vi "Archive Directory.vi"(8 "Error In":errorcluster, 11 "Folder Path":path=path "C:/Program Files (x86)/National Instruments/LabVIEW 2011/vi.lib/LabVIEW Hacker/LVH-Toolbox") -> (0 "Error Out":errorcluster)   [LabVIEW 2020, in "LMH-Toolbox.lvlib"]
doc: "Build an archive of the specified directory. The archive is created in the folder containing the directory to archive. The archive file name is the same as the directory file name with a time stamp appended."
uses:
  LMH-Toolbox.lvlib
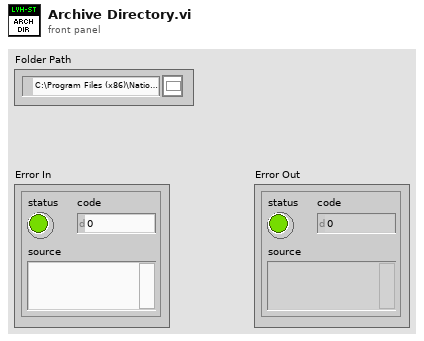
[diagram p1: front panel]
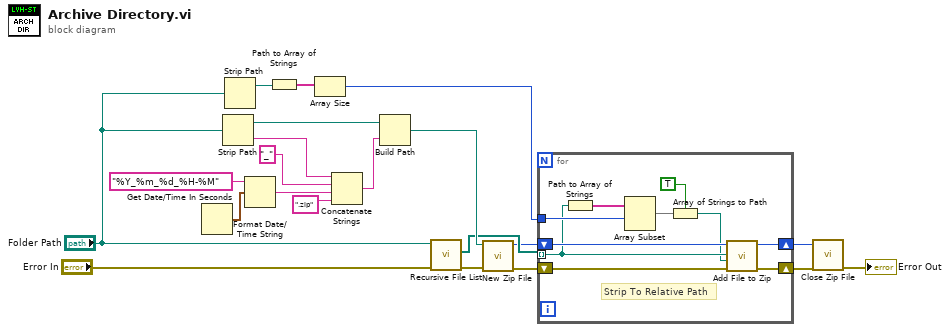
[diagram p0: block diagram]
diagram:
  n1 = Get Date/Time In Seconds() -> (seconds since 1Jan1904=w21:timestamp)
  n2 = Strip Path(path="Folder Path") -> (stripped path=w13:path, name=w12:string)
  n3 = Strip Path(path="Folder Path") -> (stripped path=w6:path)  [unwired: 1 out]
  n4 = Format Date/Time String(time format string (%c)="%Y_%m_%d_%H-%M", seconds (now)=w21) -> (date/time string=w16:string)  [unwired: 1 in]
  n5 = Path to Array of Strings(0:w6) -> (2:w5:string[])  [unwired: 1 out]
  n6 = Array Size(array=w5) -> (size(s)=w3:i32)
  n7 = Concatenate Strings(w12, "_" ("string"), w16, ".zip" ("string")) -> (w19:string)
  n8 = Build Path(base path=w13, name or relative path=w19) -> (appended path=w18:path)
  n9 = call <vilib>:"Recursive File List.vi"("error in (no error)"="Error In", "Folder Path"="Folder Path") -> ("error out"=w1:errorcluster, "All Files in Dir"=w11:path[])  [unwired: 5 in, 3 out]
  n10 = call <vilib>:"New Zip File.vi"("error in (no error)"=w1, "target"=w18) -> ("error out"=w9:errorcluster, "zip file out"=w10:i64)  [unwired: 3 in, 1 out]
  n11 = for {
    tunnel: w11 -> [w23] mode=indexing
    shift-right: [w28] -> w8
    shift-left: w9 -> [w30]
    shift-right: [w29] -> w7
    shift-left: w10 -> [w31]
    tunnel: w3 -> [w24]
    # "Strip To Relative Path"
    n12 = Path to Array of Strings(0:w23) -> (2:w27:string[])  [unwired: 1 out]
    n13 = Array Subset(array=w27, index=w24) -> (w26:string[])  [unwired: 1 in]
    n14 = Array of Strings to Path(0:w26, 1:TRUE ("relative")) -> (2:w22:path)
    n15 = call <vilib>:"Add File to Zip.vi"("error in (no error)"=w30, "destination path in zip"=w22, "source file path"=w23, "zip file in"=w31) -> ("error out"=w28:errorcluster, "zip file out"=w29:i64)  [unwired: 6 in]
  }
  n16 = call <vilib>:"Close Zip File.vi"("error in (no error)"=w8, "zip file in"=w7) -> ("error out"=→"Error Out":errorcluster)  [unwired: 5 in]
